vi "New P2P UDP Link.vi"(8 "error in (no error)":errorcluster, 9 "Port Number":u16, 10 "IP Address":string, 11 "Assert Service in":refnum<class "Assert Service.lvclass">) -> (0 "error out":errorcluster, 3 "Assert Service out":refnum<class "Assert Service.lvclass">)   [LabVIEW 2016, in "Assert API Components.lvlib" / "Assert Service.lvlib" / "Assert Service.lvclass"]
uses:
  Assert Service.lvclass
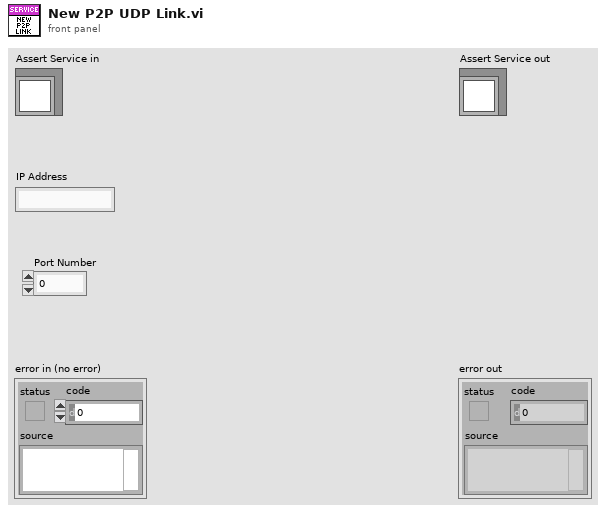
[diagram p1: front panel]
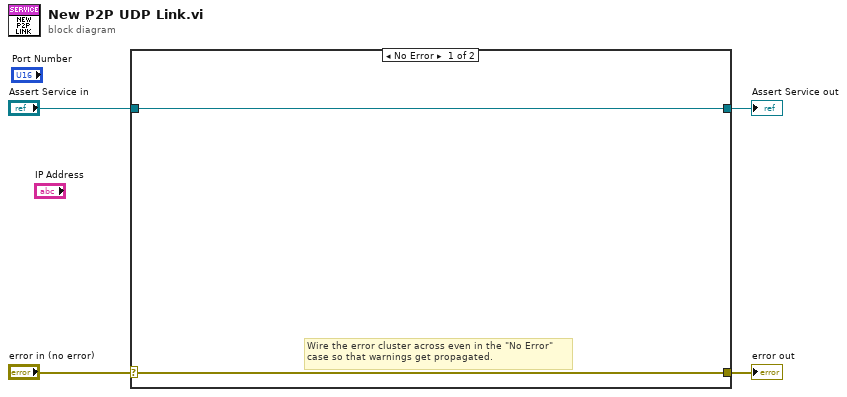
[diagram p0: block diagram]
diagram:
  n1 = case shown="No Error" "error in (no error)" {
    selector: "error in (no error)" -> [w5 w8]
    tunnel: [w5 w8] -> w3
    tunnel: [w6 w7] -> w1
    tunnel: "Assert Service in" -> [w6 w7]
    frame No Error {
      # "Wire the error cluster across even in the \"No Error\"\ncase so that warnings get propagated."
    }
    frame Error {
    }
  }
  "error out" <- w3
  "Assert Service out" <- w1
